vi "打开.vi"(8 "error in (no error)":errorcluster caption="错误输入（无错误）", 11 "路径":path) -> (0 "error out":errorcluster caption="错误输出", 3 "数据文件.lvclass":refnum<class "数据文件.lvclass">)   [LabVIEW 2021, in "数据文件.lvclass"]
doc: "本VI是为《我和LabVIEW》一书编写的示例。\n关于本书的介绍请参考网页：\nhttp://ruanqizhen.spaces.live.com/blog/cns!5852D4F797C53FB6!4310.entry"
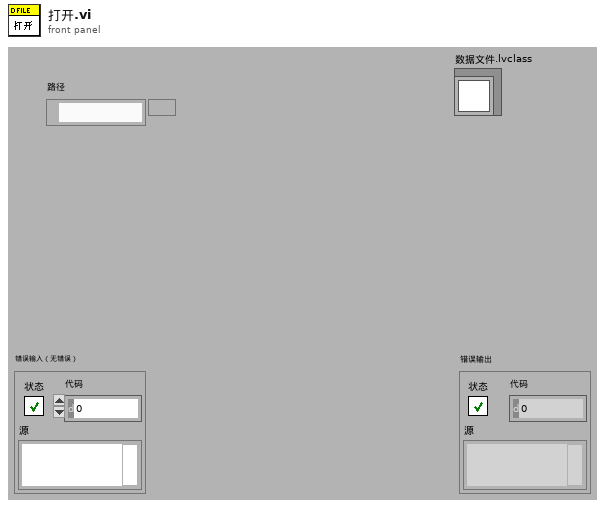
[diagram p1: front panel]
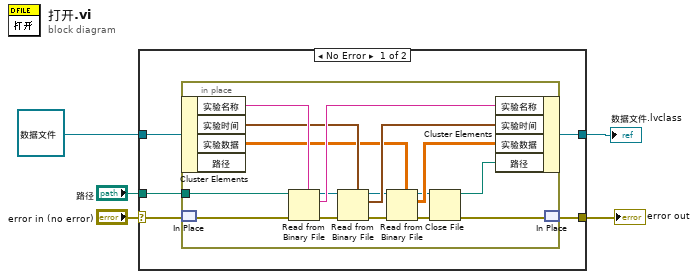
[diagram p0: block diagram]
diagram:
  n1 = case shown="No Error" "error in (no error)" {
    selector: "error in (no error)" -> [w8 w28]
    tunnel: [w7 w28] -> w4
    tunnel: [w6 w27] -> w1
    tunnel: refnum<class "数据文件.lvclass"> refnum ("数据文件.lvclass") -> [w10 w27]
    tunnel: "路径" -> [w9 _]
    frame No Error {
      n2 = in-place {
        in-place-border: w9 -> [w26]
        n3 = in-place-cluster #1(w10) -> ("实验名称"=w25:string, "实验时间"=w23:timestamp, "实验数据"=w21:dbl[][])  [unwired: 1 out]
        n4 = in-place-match #2(w8) -> (w13:errorcluster)
        n5 = Read from Binary File(5:w25, 8:w13, 11:w26) -> (0:w17:errorcluster, 2:w24:string, 3:w18:refnum<file>)  [unwired: 4 out]
        n6 = Read from Binary File(5:w23, 8:w17, 11:w18) -> (0:w16:errorcluster, 2:w22:timestamp, 3:w19:refnum<file>)  [unwired: 4 out]
        n7 = Read from Binary File(5:w21, 8:w16, 11:w19) -> (0:w14:errorcluster, 2:w20:dbl[][], 3:w15:refnum<file>)  [unwired: 4 out]
        n8 = Close File(refnum=w15, error in=w14) -> (path=w11:path, error out=w12:errorcluster)
        n9 = in-place-cluster #1("实验名称"=w24, "实验时间"=w22, "实验数据"=w20, "路径"=w11) -> (w6:refnum<class "数据文件.lvclass">)
        n10 = in-place-match #2(w12) -> (w7:errorcluster)
      }
    }
    frame Error {
    }
  }
  "error out" <- w4
  "数据文件.lvclass" <- w1
